vi "Exposure Box.vi"() -> ()   [LabVIEW 2020]
uses:
  epl-vi-lib/Utility VIs/Buttons/KCheckmarkBoolean.ctl
  epl-vi-lib/Utility VIs/Controls/KBackground Gradient/KBackground Gradient.xctl
  Typedefs/TB-Parameters.ctl
  Typedefs/TB-Analysis Parameters.ctl
  Typedefs/TB-Slack State.ctl
  Typedefs/TB-Persistent Data.ctl
  epl-vi-lib/PXI DAQ VIs/AIDI/Typedefs/AIDI-Action.ctl
  epl-vi-lib/PXI DAQ VIs/AODO/Typedefs/AODO-Action.ctl
  Typedefs/TB-State Enum.ctl
  <vilib>/Analysis/baseanly.llb/Mean (DBL).vi
  <vilib>/Analysis/5stat.llb/RMS (DBL).vi
  7ee2e33f-629f-4d1f-82d3-c59bb6443cc8.vi
  <vilib>/Analysis/NI_AALPro.lvlib
  <vilib>/Analysis/NI_AALBase.lvlib
panel:
  out "Exposure":errorcluster
  out "Crown":errorcluster
  in  "Waveform":u16(ring)=2 items=["Noise", "File", "Tone"]
  in  "dB SPL":dbl=100.0
  in  "Duration (min)":dbl=120.0
  in  "Tab Control":enum32{"Tone", "Noise", "File"}(tab)
  in  "Frequency (kHz)":dbl=8.0
  in  "High cutoff (kHz)":dbl=16.0
  in  "Low cutoff (kHz)":dbl=8.0
  in  "refWAV":path caption="Ref"
  in  "WAVfile":path
  in  "Cal Log":path=path "C:/Data/Trauma Box/Trauma Box Calibration Log.txt"
  out "Pistonphone Factor":dbl=102.0 caption="Calibrator Voltage\n(dB rms re 1 uV)"
  in  "B&K Mic Gain":dbl=20.0
  in  "Display":enum32{"Page 1", "Page 2"}(tab)
  out "ma":dbl=99.37258874088361 caption="average" format="%.1f"
  out "Starts":i32
  out "Overload 2":bool caption="Overload"
  in  "Fine Control":dbl(slide) caption="Fine Adjust (dB)" scale=-10.0..6.0
  out "Spectrum":waveform(dbl)(graph)
  out "Waveform":waveform(dbl)(graph)
  out "dB SPL rms":dbl=99.37258874088361 format="%.2f"
  out "Gauge":dbl(knob)=99.37258874088361 scale=80.0..130.0
  out "Elapsed time":string
  out "SPL History":cluster{dbl[], dbl[]}[](graph)
  out "Expected":string="Expected value = 102"
  in  "micCorrFile":path
  in  "Use mic correction":T1 caption="Apply mic frequency correction (if you're unsure, then no)"
  out "Calibration Log":string[][](table)
  out "Overload":bool
  out "Calibrator Voltage\n(dB rms re 1 uV)":dbl=-inf
  out "Pistonphone\nWaveform":dbl[](graph)
  in  "Wizard":T2(tab)
  in  "START":bool
  in  "EXIT":bool
  in  "Use previous":bool
  in  "Remeasure":bool
  in  "Pistonphone measure":bool
  in  "Next":bool
  in  "To Crown adjust":bool
  in  "Start Crown":bool
  in  "Stop Crown":bool
  in  "Start Exposure":bool
  in  "Stop Exposure":bool
  in  "Finished":bool
  in  "User ID":string
  in  "Gradient":dbl(xcontrol)
  # "dB SPL"
  # "Press START to begin\nPress EXIT to quit"
  # "Step 1 Pistonphone correction"
  # "Step 1 Pistonphone correction\n    \n--Put ref mic into pistonphone\n--Make sure B&K gain is correct"
  # "Step 2 Put microphone in cage. It's going to get loud! Close the booth door before continuing."
  # "Step 3 Adjust amplifier until SPL is correct, then hit \"Stop\" button:"
  # "Step 4: Noise Exposure\n1. Put animal(s) in cage\n2. Set duration,\n3. Press START"
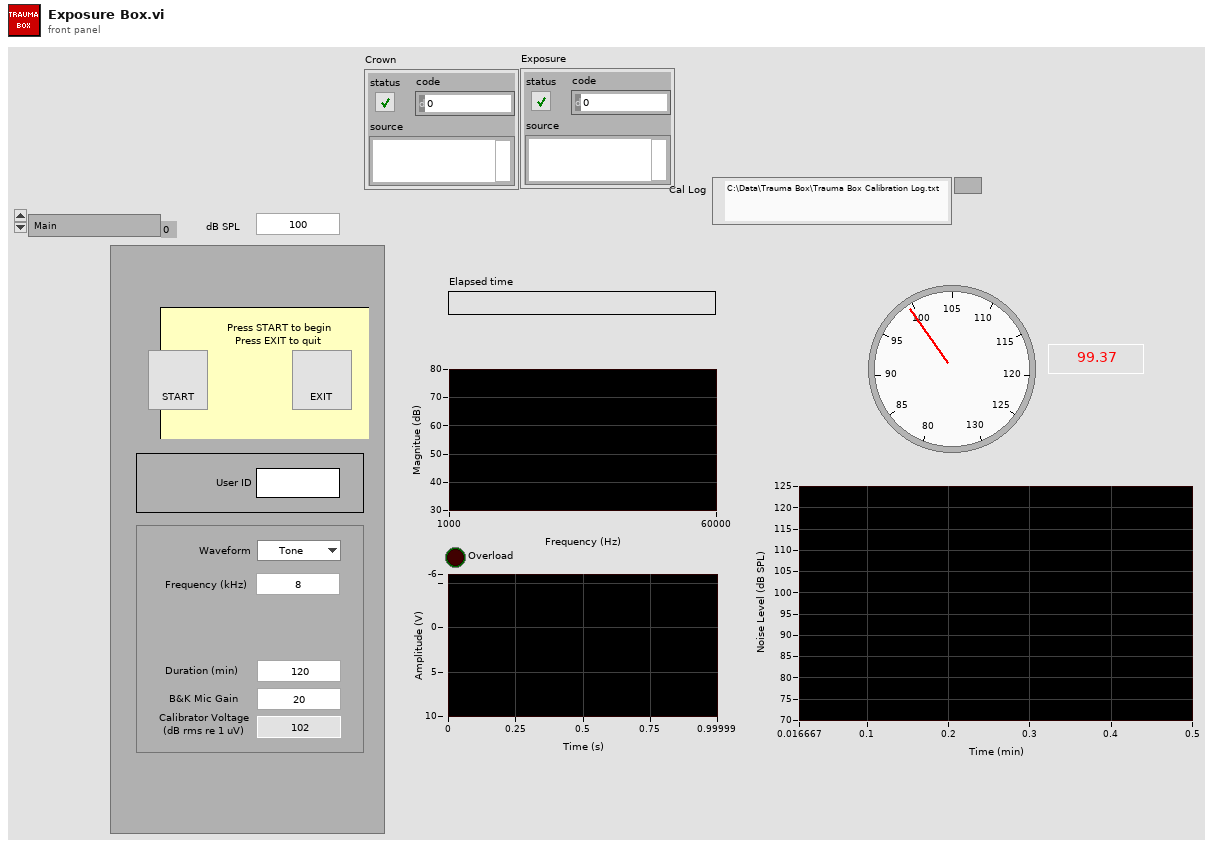
[diagram p1: front panel]
types:
  T1 = typedef "KCheckmarkBoolean.ctl" = bool
  T2 = enum32{"Main", "Pistonphone query", "Pistonphone measure", "Mic in cage", "Adjust Crown", "Animal in cage"}
  T3 = typedef "TB-Persistent Data.ctl" = cluster{"date":string, "cspd scale":dbl}
  T4 = typedef "TB-Slack State.ctl" = cluster{"access_token":string, "bot id":string, "users":cluster{"id":string, "always":bool}[], "chan id":string}
  T5 = typedef "TB-Parameters.ctl" = cluster{"Low cutoff (kHz)":dbl, "High cutoff (kHz)":dbl, "Duration (min)":dbl, "dB SPL":dbl, "Waveform":enum16{"Noise", "File", "Tone"}, "WAVfile":path, "refWav":path, "use mic correction":bool, "micCorrFile":path, "Pistonphone Level (dB SPL)":dbl, "Sampling rate (Hz)":dbl, "Buffer length (s)":dbl, "Stream mic":bool, "Fine adjust":cluster{"Max":dbl, "Min":dbl}, "Mic gain":dbl, "atten":dbl, "Allow Slack":bool, "max starts":i32, "Freq (kHz)":dbl, "Tma (s)":dbl, "Streamed":cluster{"Device":string, "Name":string}[], "Drive":string, "Speaker":string, "Mic":string, "Analysis":T6, "exposeAtten":dbl, "Digital":string}
  T6 = typedef "TB-Analysis Parameters.ctl" = cluster{"Method":enum16{"Default", "Periodogram", "Cross-spectrum"}, "resol (Hz)":dbl, "nfreq":i32, "signal":string}
  T7 = cluster{bool, "Exposure parameters":T5, "Slack":T4}
  T8 = typedef "AODO-Action.ctl" = enum16{"Configure", "Initialize", "Start", "Write", "Clean up", "Init & Start", "Config & Test", "Position", "Set AO Gains", "Zero", "Prime", "Status"}
  T9 = typedef "AIDI-Action.ctl" = enum16{"Configure", "Initialize", "Start", "Read", "Clean up", "Init & Start", "Config & Test", "Position", "Skip"}
  T10 = typedef "TB-Runtime state.ctl" = cluster{"stimfile":T11, "stream mic?":bool, "Fs":dbl, "ID":string, "micCorr":dbl[], "expose":bool, "nacq":i32, "init error":bool, "max starts":i32, "num starts":i32, "Setup":T12, "toneIndex":i32, "LastN":dbl[], "fine":dbl, "stream":refnum<file>, "names":string[], "analysis":T13}
  T11 = typedef "Sound File Refnum.ctl" = refnum<file>
  T12 = typedef "TB-Setup Log.ctl" = cluster{"Pistonphone factor":dbl, "Fine adjust":dbl, "Actual dB SPL":dbl, "CSPD factor":dbl, "Freq":dbl[], "Mag":dbl[]}
  T13 = typedef "TB-Analysis State.ctl" = cluster{"spectra/frame":i32, "pts/spectra":i32, "nfreq":i32, "imic":i32, "isig":i32, "mags":dbl[][], "method":enum16{"Default", "Periodogram", "Cross-spectrum"}, "cspd scale":dbl}
  T14 = typedef "TB-Stimulus State.ctl" = cluster{"filelen":i32, "stimfile":T11, "stimfile?":bool, "Fs":dbl, "Npts":i32, "stimfileend":bool, "atten":dbl, "SigMan":refnum<class "SignalManager.lvclass">, "nbuf":i32, "expose?":bool}
  T15 = typedef "TB-Log.ctl" = cluster{"Slack":T4, "entries":string[]}
  T16 = typedef "TB-Mic Queue.ctl" = refnum<queue>
  T17 = typedef "TB-State Enum.ctl" = enum16{"Main", "Pistonphone query", "Pistonphone measure", "Mic in cage", "Adjust Crown", "Animal in cage"}
  T18 = enum8{"Enabled", "Disabled", "Disabled and Grayed Out"}
  T19 = cluster{"notification":bool, "Parameters out":T5, "Slack":T4}
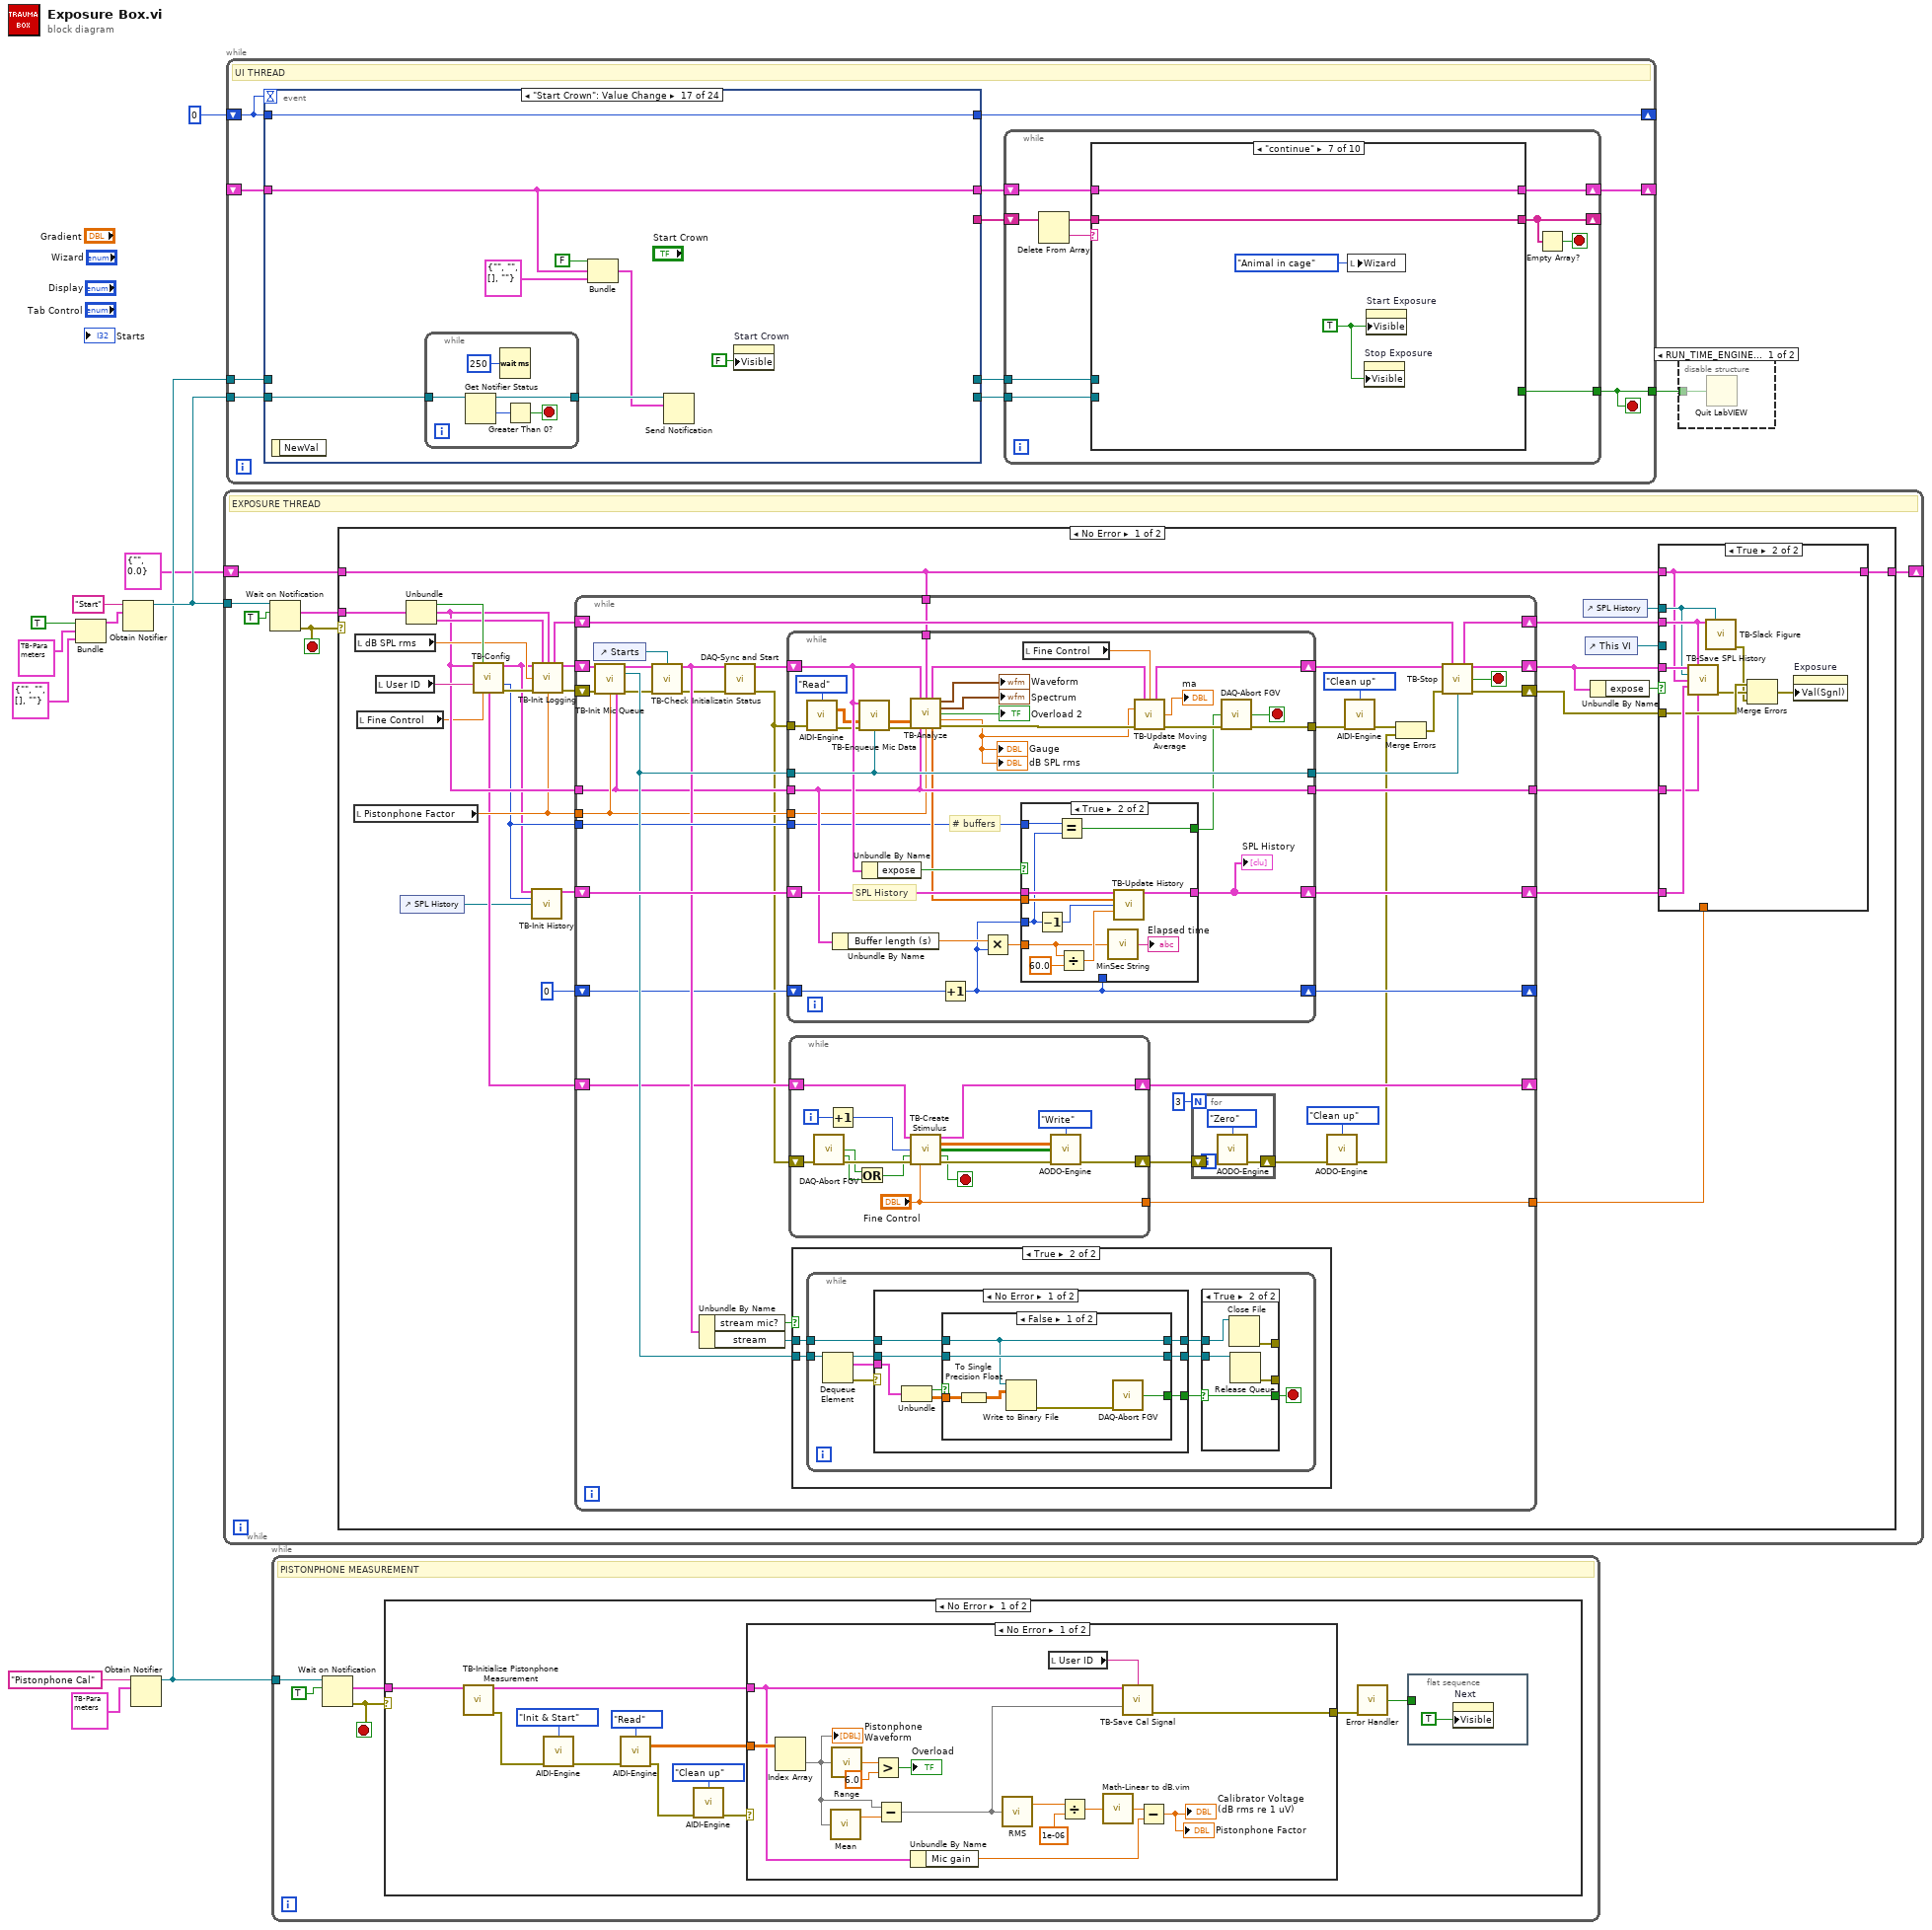
[diagram p0: block diagram]
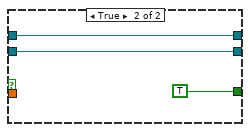
[diagram p5: hidden frame]
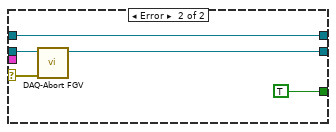
[diagram p6: hidden frame]
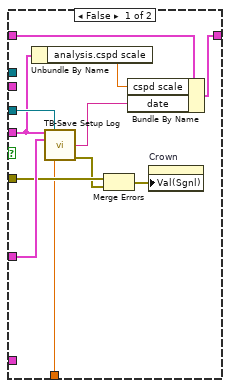
[diagram p7: hidden frame]
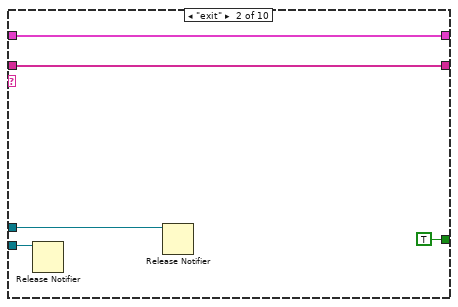
[diagram p10: hidden frame]
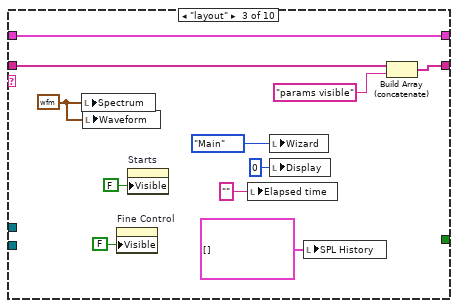
[diagram p11: hidden frame]
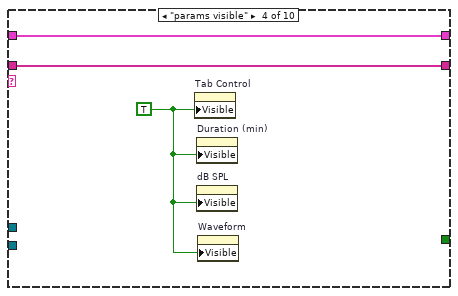
[diagram p12: hidden frame]
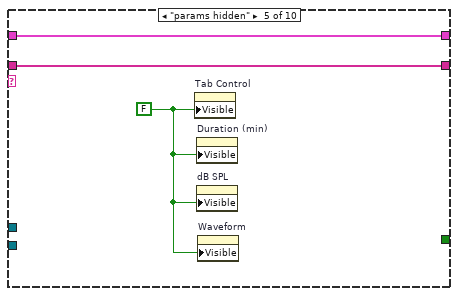
[diagram p13: hidden frame]
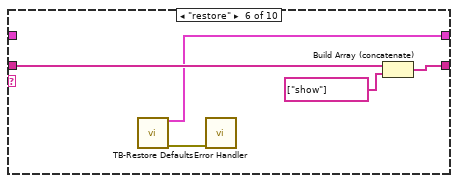
[diagram p14: hidden frame]
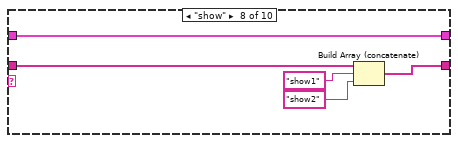
[diagram p15: hidden frame]
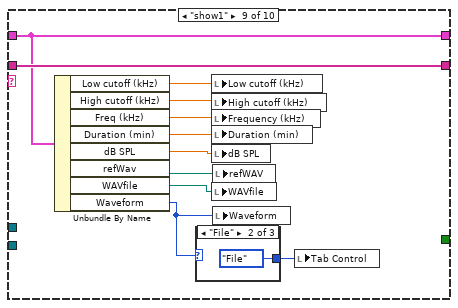
[diagram p16: hidden frame]
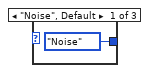
[diagram p17: hidden frame]
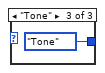
[diagram p18: hidden frame]
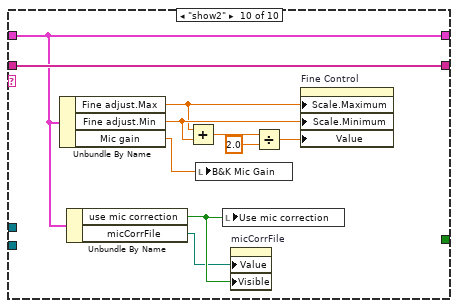
[diagram p19: hidden frame]
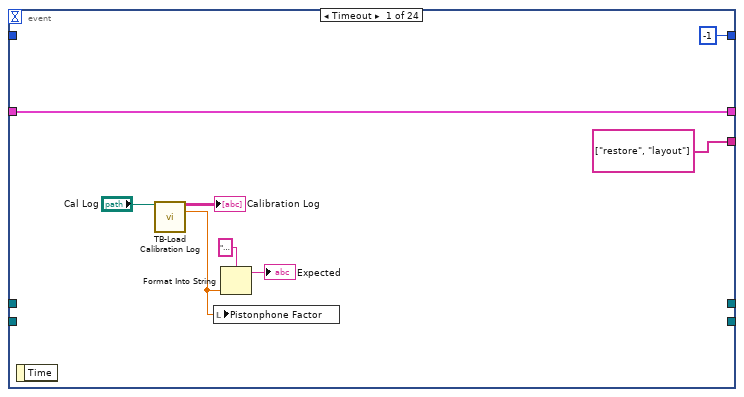
[diagram p20: hidden frame]
diagram:
  n1 = Bundle(TRUE, "Exposure parameters"=T5 {"Low cutoff (kHz)"=0.0, "High cutoff (kHz)"=0.0, "Duration (min)"=0.0, "dB SPL"=0.0, "Waveform"=enum."Noise", "WAVfile"=path "", "refWav"=path "", "use mic correction"=FALSE, "micCorrFile"=path "", "Pistonphone Level (dB SPL)"=0.0, "Sampling rate (Hz)"=0.0, "Buffer length (s)"=0.0, "Stream mic"=FALSE, "Fine adjust"={"Max"=0.0, "Min"=0.0}, "Mic gain"=0.0, "atten"=0.0, "Allow Slack"=FALSE, "max starts"=0, "Freq (kHz)"=8.0, "Tma (s)"=0.0, "Streamed"=[], "Drive"="", "Speaker"="", "Mic"="", "Analysis"={"Method"=enum."Default", "resol (Hz)"=0.0, "nfreq"=0, "signal"=""}, "exposeAtten"=0.0, "Digital"=""}, "Slack"=T4 {"access_token"="", "bot id"="", "users"=[], "chan id"=""}) -> (w4:T7)  [unwired: 1 in]
  n2 = Obtain Notifier(name (unnamed)="Start", notification data type=w4) -> (notifier out=w12:refnum<notifier>)  [unwired: 2 in, 2 out]
  n3 = Obtain Notifier(name (unnamed)="Pistonphone Cal", notification data type=T5 {"Low cutoff (kHz)"=114.0, "High cutoff (kHz)"=100000.0, "Duration (min)"=1.0, "dB SPL"=100.0, "Waveform"=enum."Noise", "WAVfile"=path "", "refWav"=path "", "use mic correction"=FALSE, "micCorrFile"=path "", "Pistonphone Level (dB SPL)"=0.0, "Sampling rate (Hz)"=0.0, "Buffer length (s)"=0.0, "Stream mic"=FALSE, "Fine adjust"={"Max"=0.0, "Min"=0.0}, "Mic gain"=0.0, "atten"=0.0, "Allow Slack"=FALSE, "max starts"=0, "Freq (kHz)"=8.0, "Tma (s)"=0.0, "Streamed"=[], "Drive"="", "Speaker"="", "Mic"="", "Analysis"={"Method"=enum."Default", "resol (Hz)"=0.0, "nfreq"=0, "signal"=""}, "exposeAtten"=0.0, "Digital"=""} ("Exposure parameters")) -> (notifier out=w8:refnum<notifier>)  [unwired: 2 in, 2 out]
  n4 = while {
    tunnel: w12 -> [w17]
    shift-right: [w13] -> _
    shift-left: T3 {"date"="", "cspd scale"=0.0} ("persist") -> [w14]
    stop <- w16 stop-if-true
    # "EXPOSURE THREAD"
    n5 = Wait on Notification(notifier=w17, ignore previous (F)=TRUE) -> (notification=w15:T7, error out=w16:errorcluster)  [unwired: 2 in, 2 out]
    n6 = case shown="No Error" w16 {
      tunnel: w15 -> [w47 _]
      tunnel: w14 -> [w19 w210]
      tunnel: [w20 w210] -> w13
      frame No Error {
        n7 = local read "Pistonphone Factor"() -> (w29:dbl)
        n8 = local read "dB SPL rms"() -> (w37:dbl)
        n9 = local read "Fine Control"() -> (w21:dbl)
        n10 = local read "User ID"() -> (w45:string)
        n11 = control-ref of="SPL History"() -> (w25:refnum<vi>)
        n12 = Unbundle(w47) -> (w46:bool, "Exposure parameters"=w36:T5, "Slack"=w39:T4)
        n13 = call "TB-Config.vi"("Params"=w36, "Exposure?"=w46, "ID"=w45, "Fine adjust (dB)"=w21) -> ("state"=w23:T10, "Num Buffers"=w24:i32, "stimulus state"=w26:T14, "error out"=w41:errorcluster)  [unwired: 8 in]
        n14 = call "TB-Init History.vi"("state"=w23, "Num Buffers"=w24, "XYGraph in"=w25) -> ("history"=w22:cluster{dbl[], dbl[]}[])  [unwired: 12 in]
        n15 = call "TB-Init Logging.vi"("state in"=w23, "Slack"=w39, "Params"=w36, "Level"=w37, "error in (no error)"=w41, "Pistonphone factor"=w29) -> ("Log"=w34:T15, "state out"=w38:T10, "error out"=w40:errorcluster)  [unwired: 7 in]
        n16 = while {
          tunnel: w29 -> [w61]
          tunnel: w24 -> [w81]
          tunnel: w36 -> [w60]
          shift-right: [w82] -> w44
          shift-left: w22 -> [w86]
          shift-right: [w78] -> w42
          shift-left: w40 -> [w77]
          shift-right: [w75] -> w35
          shift-left: w38 -> [w76]
          shift-right: [w73] -> w33
          shift-left: w34 -> [w74]
          shift-right: [w67] -> _
          shift-left: 0 -> [w68]
          shift-right: [w65] -> _
          shift-left: w26 -> [w64]
          tunnel: [w63] -> w30
          tunnel: [w62] -> w28
          tunnel: w19 -> [w50]
          stop <- w69 stop-if-true
          n17 = control-ref of="Starts"() -> (w66:refnum<vi>)
          n18 = call "TB-Init Mic Queue.vi"("state in"=w76, "error in (no error)"=w77, "Pistonphone factor"=w61, "Exposure parameters"=w60) -> ("state out"=w71:T10, "mic queue"=w85:T16, "error out"=w72:errorcluster)  [unwired: 9 in]
          n19 = call "TB-Check Initializatin Status.vi"("state in"=w71, "Starts"=w66, "error in (no error)"=w72) -> ("state out"=w70:T10, "error out"=w53:errorcluster)  [unwired: 11 in]
          n20 = Unbundle By Name(w70) -> ("stream mic?"=w80:bool, "stream"=w84:refnum<file>)
          n21 = call "DAQ-Sync and Start.vi"("error in (no error)"=w53) -> ("error out"=w52:errorcluster)  [unwired: 14 in]
          n22 = while {
            tunnel: w81 -> [w92]
            shift-right: [w118] -> w82
            shift-left: w86 -> [w120]
            tunnel: w61 -> [w99]
            tunnel: w60 -> [w107]
            tunnel: w85 -> [w113]
            tunnel: [w113] -> w83
            shift-right: [w103] -> w79
            shift-left: w70 -> [w110]
            tunnel: [w111] -> w55
            shift-right: [w93] -> w67
            shift-left: w68 -> [w108]
            tunnel: [w107] -> w63
            tunnel: w52 -> [w94]
            tunnel: w50 -> [w90]
            stop <- w112 stop-if-true
            # "# buffers"
            # "SPL History"
            n23 = call "AIDI-Engine.vi"("Action"=AIDI-Action."Read", "error in (no error)"=w94) -> ("AI"=w96:dbl[][], "error out"=w97:errorcluster)  [unwired: 8 in, 4 out]
            n24 = Unbundle By Name(w107) -> ("Buffer length (s)"=w116:dbl)
            n25 = call "TB-Enqueue Mic Data.vi"("state thru"=w110, "AI Waveforms in"=w96, "error in (no error)"=w97, "Queue in"=w113) -> ("AI Waveforms thru"=w115:dbl[][], "error out"=w114:errorcluster)  [unwired: 10 in]
            n26 = Unbundle By Name(w110) -> ("expose"=w109:bool)
            n27 = call "TB-Analyze.vi"("state in"=w110, "persist"=w90, "AI Waveforms"=w115, "error in (no error)"=w114, "Exposure parameters"=w107, "Pistonphone Factor"=w99) -> ("state out"=w104:T10, "waveform"=→"Waveform":waveform(dbl), "spectrum"=→"Spectrum":waveform(dbl), "Overload"=→"Overload 2":bool, "Cal SPL"=w101:dbl, "history values"=w98:dbl[], "error out"=w106:errorcluster)  [unwired: 3 in]
            "Gauge" <- w101
            "dB SPL rms" <- w101
            n28 = Increment(x=w108) -> (x+1=w93:i32)
            n29 = Multiply(x=w116, y=w93) -> (x*y=w121:dbl)
            n30 = case shown="True" w109 {
              tunnel: w121 -> [_ w127]
              tunnel: w120 -> [w123 w132]
              tunnel: [w123 w131] -> w118
              tunnel: w98 -> [_ w130]
              tunnel: w93 -> [_ w125]
              tunnel: w93 -> [_ _]
              tunnel: w92 -> [_ w126]
              tunnel: [_ w124] -> w91
              frame False {
              }
              frame True {
                n31 = Decrement(x=w125) -> (x-1=w129:i32)
                n32 = Equal?(x=w126, y=w125) -> (x = y?=w124:bool)
                n33 = Divide(x=w127, y=60.0) -> (x/y=w128:dbl)
                n34 = call "MinSec String.vi"("Seconds"=w127) -> ("MinSec string"=→"Elapsed time":string)
                n35 = call "TB-Update History.vi"("history in"=w132, "history values"=w130, "Index"=w129, "Time"=w128) -> ("history out"=w131:cluster{dbl[], dbl[]}[])  [unwired: 11 in]
              }
            }
            "SPL History" <- w118
            n36 = local read "Fine Control"() -> (w100:dbl)
            n37 = call "TB-Update Moving Average.vi"("state in"=w104, "fine"=w100, "SPL"=w101, "error in (no error)"=w106) -> ("state out"=w103:T10, "moving average"=→"ma":dbl, "error out"=w105:errorcluster)  [unwired: 9 in]
            n38 = call "DAQ-Abort FGV.vi"("Finished"=w91, "error in (no error)"=w105) -> ("Stop"=w112:bool, "Errors"=w111:errorcluster)  [unwired: 11 in, 1 out]
          }
          n39 = while {
            shift-right: [w148] -> w51
            shift-left: w52 -> [w143]
            shift-right: [w146] -> w65
            shift-left: w64 -> [w147]
            tunnel: ["Fine Control"] -> w62
            i -> [w144]
            stop <- w140 stop-if-true
            n40 = call "DAQ-Abort FGV.vi"("error in (no error)"=w143) -> ("Stop"=w139:bool, "Was aborted"=w138:bool, "Errors"=w142:errorcluster)  [unwired: 12 in]
            n41 = Increment(x=w144) -> (x+1=w141:i32)
            n42 = Or(x=w139, y=w138) -> (x .or. y?=w137:bool)
            n43 = call "TB-Create Stimulus.vi"("state"=w147, "Num"=w141, "quit"=w137, "error in (no error)"=w142, "Fine adjust (dB)"="Fine Control") -> ("state out"=w146:T14, "stimulus"=w136:dbl[][], "digital"=w135:bool[][], "finished"=w140:bool, "error out"=w149:errorcluster)  [unwired: 6 in]
            n44 = call "AODO-Engine.vi"("Action"=AODO-Action."Write", "AO"=w136, "DO"=w135, "error in (no error)"=w149) -> ("error out"=w148:errorcluster)  [unwired: 6 in, 5 out]
          }
          n45 = case shown="True" w80 {
            tunnel: w85 -> [_ w152]
            tunnel: w84 -> [_ w151]
            frame False {
            }
            frame True {
              n46 = while {
                tunnel: w152 -> [w161]
                tunnel: w151 -> [w155]
                stop <- w156 stop-if-true
                n47 = Dequeue Element(queue=w161) -> (queue out=w158:T16, element=w159:cluster{bool, dbl[][]}, error out=w160:errorcluster)  [unwired: 2 in, 1 out]
                n48 = case shown="No Error" w160 {
                  selector: w160 -> [_ w185]
                  tunnel: w159 -> [w175 _]
                  tunnel: [w173 TRUE ("status")] -> w157
                  tunnel: w158 -> [w171 w186]
                  tunnel: w155 -> [w170 w187]
                  tunnel: [w169 w187] -> w154
                  tunnel: [w168 w186] -> w153
                  frame No Error {
                    n49 = Unbundle(w175) -> (w174:bool, w172:dbl[][])
                    n50 = case shown="False" w174 {
                      tunnel: [w180 TRUE ("status")] -> w173
                      tunnel: w172 -> [w177 _]
                      tunnel: w171 -> [w181 w182]
                      tunnel: w170 -> [w179 w183]
                      tunnel: [w179 w183] -> w169
                      tunnel: [w181 w182] -> w168
                      frame False {
                        n51 = To Single Precision Float(number=w177) -> (single precision float=w176:sgl[][])
                        n52 = Write to Binary File(file (use dialog)=w179, data=w176) -> (error out=w178:errorcluster)  [unwired: 4 in, 2 out]
                        n53 = call "DAQ-Abort FGV.vi"("error in (no error)"=w178) -> ("Stop"=w180:bool)  [unwired: 12 in, 2 out]
                      }
                      frame True {
                      }
                    }
                  }
                  frame Error {
                    n54 = call "DAQ-Abort FGV.vi"("error in (no error)"=w185) -> ()  [unwired: 12 in, 3 out]
                  }
                }
                n55 = case shown="True" w157 {
                  selector: w157 -> [w162 w167]
                  tunnel: [w162 w167] -> w156
                  tunnel: w154 -> [_ w164]
                  tunnel: w153 -> [_ w166]
                  tunnel: [_ w165] -> _
                  tunnel: [_ w163] -> _
                  frame False {
                  }
                  frame True {
                    n56 = Close File(refnum=w164) -> (error out=w163:errorcluster)  [unwired: 1 in, 1 out]
                    n57 = Release Queue(queue=w166) -> (error out=w165:errorcluster)  [unwired: 2 in, 2 out]
                  }
                }
              }
            }
          }
          n58 = for {
            N: 3 -> [_]
            shift-right: [w87] -> w49
            shift-left: w51 -> [w89]
            n59 = call "AODO-Engine.vi"("Action"=AODO-Action."Zero", "error in (no error)"=w89) -> ("error out"=w87:errorcluster)  [unwired: 8 in, 5 out]
          }
          n60 = call "AODO-Engine.vi"("Action"=AODO-Action."Clean up", "error in (no error)"=w49) -> ("error out"=w57:errorcluster)  [unwired: 8 in, 5 out]
          n61 = call "AIDI-Engine.vi"("Action"=AIDI-Action."Clean up", "error in (no error)"=w55) -> ("error out"=w56:errorcluster)  [unwired: 8 in, 5 out]
          n62 = Merge Errors(w56, w57) -> (w54:errorcluster)
          n63 = call "TB-Stop.vi"("state in"=w79, "Log in"=w74, "error in (no error)"=w54, "Queue in"=w83) -> ("Log out"=w73:T15, "state out"=w75:T10, "Finished"=w69:bool, "error out"=w78:errorcluster)  [unwired: 8 in]
        }
        n64 = control-ref of="SPL History"() -> (w31:refnum<vi>)
        n65 = control-ref of="This VI"() -> (w27:refnum<vi>)
        n66 = Unbundle By Name(w35) -> ("expose"=w43:bool)
        n67 = case shown="True" w43 {
          tunnel: w44 -> [_ w209]
          tunnel: w35 -> [w190 w208]
          tunnel: w42 -> [w198 w207]
          tunnel: w33 -> [_ w203]
          tunnel: w31 -> [_ w202]
          tunnel: w30 -> [w199 w201]
          tunnel: w28 -> [w195 _]
          tunnel: w27 -> [w194 _]
          tunnel: w19 -> [w193 w200]
          tunnel: [w191 w200] -> w20
          frame False {
            n68 = Unbundle By Name(w190) -> ("analysis.cspd scale"=w189:dbl)
            n69 = call "TB-Save Setup Log.vi"("State"=w190, "VI ref"=w194, "Exposure parameters"=w199, "Fine Control"=w195) -> ("date/time string"=w192:string, "error out"=w196:errorcluster)  [unwired: 10 in]
            n70 = Merge Errors(w198, w196) -> (w197:errorcluster)
            n71 = Bundle By Name(cluster=w193, "cspd scale"=w189, "date"=w192) -> (w191:T3)
            n72 = property on="Crown" class="Clust (strict)"("Val(Sgnl)"=w197) -> ()  [unwired: 2 in, 2 out]
          }
          frame True {
            n73 = call "TB-Save SPL History.vi"("state"=w208, "Log in"=w203, "XYGraph in"=w202, "persistent"=w200, "history"=w209, "Exposure parameters"=w201) -> ("error out"=w205:errorcluster)  [unwired: 9 in]
            n74 = call "TB-Slack Figure.vi"("Log"=w203, "XYGraph in"=w202) -> ("error out"=w204:errorcluster)  [unwired: 13 in]
            n75 = Merge Errors(w207, w205, w204) -> (w206:errorcluster)
            n76 = property on="Exposure" class="Clust (strict)"("Val(Sgnl)"=w206) -> ()  [unwired: 2 in, 2 out]
          }
        }
      }
      frame Error {
      }
    }
  }
  n77 = while {
    tunnel: w12 -> [w221]
    shift-right: [w220] -> _
    shift-left: 0 -> [w217]
    tunnel: w8 -> [w219]
    tunnel: [w211] -> w7
    shift-right: [w212] -> _
    shift-left: _ -> [w218]
    stop <- w211 stop-if-true
    # "UI THREAD"
    n78 = event shown="[16] \"Start Crown\": Value Change" {
      selector: _ -> [_ _ _ _ _ _ _ _ _ _ _ _ _ _ _ _ _ _ _ _ _ _ _ _]
      dyn-events: _ -> [_ _ _ _ _ _ _ _ _ _ _ _ _ _ _ _ _ _ _ _ _ _ _ _]
      timeout: w217 -> [_ _ _ _ _ _ _ _ _ _ _ _ _ _ _ _ _ _ _ _ _ _ _ _]
      tunnel: w221 -> [_ w302 w309 _ _ _ _ _ _ _ _ _ _ _ _ w411 w419 _ w453 _ _ w474 _ _]
      tunnel: [_ w302 w309 _ _ _ _ _ _ _ _ _ _ _ _ _ _ _ _ _ _ w474 _ _] -> w214
      tunnel: [-1 w305 w313 w340 w346 w352 w355 w360 w368 w369 w374 w381 w385 w391 w394 w404 w415 w428 w436 w465 w467 w471 w478 w484] -> w220
      tunnel: w219 -> [_ w303 w310 _ _ _ _ _ _ _ _ _ _ w392 _ _ _ _ _ _ _ w473 _ _]
      tunnel: [_ w303 w310 _ _ _ _ _ _ _ _ _ _ _ _ _ _ _ _ _ _ w473 _ _] -> w215
      tunnel: [w298 w306 w311 w341 w349 w353 w358 w363 w366 w372 w375 w382 w386 w390 w395 w401 w416 w429 w434 w466 w468 w472 w477 w483] -> w213
      tunnel: w218 -> [w298 w306 w314 w342 w350 w354 w359 w364 w367 w373 w375 w382 w386 w390 w395 w401 w416 w429 w434 w466 w468 w472 w477 w483]
      tunnel: w217 -> [_ w305 w313 w340 w346 w352 w355 w360 w368 w369 w374 w381 w385 w391 w394 w404 w415 w428 w436 w465 w467 w471 w478 w484]
      tunnel: [string[] ["restore", "layout"] string[] ["exit"] w312 _ _ _ _ _ _ _ _ _ string[] ["params hidden"] _ string[] ["params visible"] _ _ _ _ _ _ string[] ["exit"] _ _] -> w216
      event Timeout {
        n79 = event-data() -> ()  [unwired: 1 in, 1 out]
        n80 = call "TB-Load Calibration Log.vi"("Cal Log"="Cal Log") -> ("Log"=→"Calibration Log":string[][], "mean value"=w296:dbl)  [unwired: 13 in]
        n81 = local write "Pistonphone Factor"(w296) -> ()
        n82 = Format Into String(format string="Expected value = %d", w296) -> (resulting string=→"Expected":string)  [unwired: 2 in, 1 out]
      }
      event Panel Close? {
        n83 = event-data() -> ()  [unwired: 1 in, 1 out]
        n84 = event-data("Discard?"=TRUE) -> ()  [unwired: 1 in, 1 out]
      }
      event Menu Selection (User) {
        n85 = event-data() -> ("ItemTag"=w315:string)  [unwired: 1 in]
        n86 = case shown="\"mmFileContinue\"" w315 {
          tunnel: [_ _ w324 _ _ _ _] -> w308
          tunnel: w314 -> [w316 w317 w321 w330 w332 w334 w336]
          tunnel: [w316 w317 w320 w330 w332 w334 w337] -> w311
          tunnel: [_ string[] ["restore"] _ string[] ["restore", "layout"] string[] ["continue"] string[] ["exit"] _] -> w312
          frame "", Default {
          }
          frame "mmFileRestore" {
          }
          frame "mmFileSave" {
            n87 = property on="Fine Control" class="Slide (strict)"() -> ("Scale.Maximum"=w323:dbl, "Scale.Minimum"=w322:dbl)  [unwired: 2 in, 2 out]
            n88 = Bundle By Name(cluster=w321, "Fine adjust.Max"=w323, "Fine adjust.Min"=w322) -> (w320:T5)
            n89 = call "Default Config File Path.vi"() -> ("Default config file name"=w326:path)
            n90 = call "Write Anything.vi"("Section Name (Name of \"Anything\")"="Params" ("Section Name (Name of \"Anything\")"), "Anything"=w320, "Path (dialog)"=w326) -> ("Error Out"=w325:errorcluster)  [unwired: 7 in, 1 out]
            n91 = case shown="No Error" w325 {
              selector: w325 -> [_ w328]
              tunnel: [_ w328] -> w324
              frame No Error {
                n92 = One Button Dialog(message="Defaults saved.") -> ()  [unwired: 1 in, 1 out]
              }
              frame Error {
              }
            }
          }
          frame "mmFileRestart" {
          }
          frame "mmFileContinue" {
          }
          frame "mmFileExit" {
          }
          frame "mmEditOptions" {
            n93 = control-ref of="This VI"() -> (w335:refnum<vi>)
            n94 = call "TB-Options Dialog.vi"("Parameters in"=w336, "Parent VI"=w335) -> ("Parameters out"=w337:T5)  [unwired: 12 in, 1 out]
          }
        }
        n95 = call "Error Handler.vi"("error in (no error)"=w308) -> ()  [unwired: 12 in, 3 out]
      }
      event "Waveform": Value Change {
        n96 = event-data() -> ()  [unwired: 1 in, 1 out]
        n97 = case shown="1" "Waveform" {
          tunnel: [enum32{"Tone", "Noise", "File"}."Noise" ("Tab Control") enum32{"Tone", "Noise", "File"}."File" ("Tab Control") enum32{"Tone", "Noise", "File"}."Tone" ("Tab Control")] -> w339
          frame 0, Default {
          }
          frame 1 {
          }
          frame 2 {
          }
        }
        n98 = local write "Tab Control"(w339) -> ()
        n99 = Bundle By Name(cluster=w342, "Waveform"="Waveform") -> (w341:T5)
      }
      event "Low cutoff (kHz)", "High cutoff (kHz)": Value Change {
        n100 = event-data() -> ()  [unwired: 1 in, 1 out]
        n101 = Bundle By Name(cluster=w350, "Low cutoff (kHz)"="Low cutoff (kHz)", "High cutoff (kHz)"="High cutoff (kHz)") -> (w349:T5)
      }
      event "Frequency (kHz)": Value Change {
        n102 = event-data() -> ()  [unwired: 1 in, 1 out]
        n103 = Bundle By Name(cluster=w354, "Freq (kHz)"="Frequency (kHz)") -> (w353:T5)
      }
      event "WAVfile", "refWAV": Value Change {
        n104 = event-data() -> ()  [unwired: 1 in, 1 out]
        n105 = Bundle By Name(cluster=w359, "WAVfile"="WAVfile", "refWav"="refWAV") -> (w358:T5)
      }
      event "micCorrFile": Value Change {
        n106 = event-data() -> ()  [unwired: 1 in, 1 out]
        n107 = Bundle By Name(cluster=w364, "use mic correction"="Use mic correction", "micCorrFile"="micCorrFile") -> (w363:T5)
        n108 = property on="micCorrFile" class="Path"("Visible"="Use mic correction") -> ()  [unwired: 2 in, 2 out]
      }
      event "B&K Mic Gain": Value Change {
        n109 = event-data() -> ()  [unwired: 1 in, 1 out]
        n110 = Bundle By Name(cluster=w367, "Mic gain"="B&K Mic Gain") -> (w366:T5)
      }
      event "Duration (min)", "dB SPL": Value Change {
        n111 = event-data() -> ()  [unwired: 1 in, 1 out]
        n112 = Bundle By Name(cluster=w373, "Duration (min)"="Duration (min)", "dB SPL"="dB SPL") -> (w372:T5)
      }
      event "START": Value Change {
        n113 = event-data() -> ()  [unwired: 1 in, 1 out]
        n114 = Empty String/Path?(string/path="User ID") -> (empty?=w376:bool)
        n115 = case shown="False" w376 {
          frame False {
            n116 = property on="Starts" class="DigNum (strict)"("Visible"=FALSE) -> ()  [unwired: 2 in, 2 out]
            n117 = local write "Wizard"(TB-State_Enum."Pistonphone query" ("State")) -> ()
          }
          frame True {
            n118 = One Button Dialog(message="Please enter a User ID (for bookkeeping purposes).") -> ()  [unwired: 1 in, 1 out]
          }
        }
      }
      event "Use previous": Value Change {
        n119 = event-data() -> ()  [unwired: 1 in, 1 out]
        n120 = local write "Wizard"(TB-State_Enum."Mic in cage" ("State")) -> ()
      }
      event "Remeasure": Value Change {
        n121 = event-data() -> ()  [unwired: 1 in, 1 out]
        n122 = property on="Next" class="Bool"("Visible"=FALSE) -> ()  [unwired: 2 in, 2 out]
        n123 = local write "Display"(1) -> ()
        n124 = local write "Wizard"(TB-State_Enum."Pistonphone measure" ("State")) -> ()
      }
      event "Pistonphone measure": Value Change {
        n125 = event-data() -> ()  [unwired: 1 in, 1 out]
        n126 = Send Notification(notification=w390, notifier=w392) -> ()  [unwired: 1 in, 2 out]
      }
      event "Next": Value Change {
        n127 = event-data() -> ()  [unwired: 1 in, 1 out]
        n128 = local write "Wizard"(TB-State_Enum."Mic in cage" ("State")) -> ()
        n129 = local write "Display"(0) -> ()
      }
      event "To Crown adjust": Value Change {
        n130 = event-data() -> ()  [unwired: 1 in, 1 out]
        n131 = property on="Fine Control" class="Slide (strict)"("Visible"=TRUE, "Value"=0.0 ("Fine Control")) -> (error out=w406:errorcluster)  [unwired: 2 in, 1 out]
        n132 = local write "Elapsed time"("" ("Elapsed time")) -> ()
        n133 = local write "Wizard"(TB-State_Enum."Adjust Crown" ("State")) -> ()
        n134 = Bundle("notification"=FALSE, "Parameters out"=w401, "Slack"=T4 {"access_token"="", "bot id"="", "users"=[], "chan id"=""}) -> (w403:T19)  [unwired: 1 in]
        n135 = Send Notification(notification=w403, notifier=w411, error in (no error)=w406) -> ()  [unwired: 2 out]
        n136 = property on="Start Crown" class="Bool"("Visible"=FALSE) -> ()  [unwired: 2 in, 2 out]
        n137 = property on="Stop Crown" class="Bool"("DisabledEnum"=T18."Enabled" ("Disabled")) -> ()  [unwired: 2 in, 2 out]
        n138 = Unbundle By Name(w401) -> ("Tma (s)"=w400:dbl)
        n139 = Greater Than 0?(x=w400) -> (x > 0?=w399:bool)
        n140 = property on="ma" class="DigNum (strict)"("Visible"=w399) -> ()  [unwired: 2 in, 2 out]
      }
      event "Start Crown": Value Change {
        n141 = event-data() -> ()  [unwired: 1 in, 1 out]
        n142 = while {
          tunnel: w419 -> [w425]
          tunnel: [w421] -> w418
          stop <- w423 stop-if-true
          n143 = Get Notifier Status(notifier=w425) -> (notifier out=w421:refnum<notifier>, # waiting=w424:i32)  [unwired: 1 in, 3 out]
          n144 = Wait (ms)(milliseconds to wait=u32 250) -> ()  [unwired: 1 out]
          n145 = Greater Than 0?(x=w424) -> (x > 0?=w423:bool)
        }
        n146 = Bundle("notification"=FALSE, "Parameters out"=w416, "Slack"=T4 {"access_token"="", "bot id"="", "users"=[], "chan id"=""}) -> (w414:T19)  [unwired: 1 in]
        n147 = Send Notification(notification=w414, notifier=w418) -> ()  [unwired: 1 in, 2 out]
        n148 = property on="Start Crown" class="Bool"("Visible"=FALSE) -> ()  [unwired: 2 in, 2 out]
      }
      event "Stop Crown": Value Change {
        n149 = event-data() -> ()  [unwired: 1 in, 1 out]
        n150 = property on="Stop Crown" class="Bool"("DisabledEnum"=T18."Disabled and Grayed Out" ("Disabled")) -> ()  [unwired: 2 in, 2 out]
        n151 = call "DAQ-Abort FGV.vi"("Action"=enum16{"Default", "Init", "Abort", "1st error"}."Abort") -> ()  [unwired: 12 in, 3 out]
      }
      event "Start Exposure": Value Change {
        n152 = event-data() -> ("CtlRef"=w431:refnum<vi>)  [unwired: 1 in]
        n153 = local read "Pistonphone Factor"() -> (w447:dbl)
        n154 = Get Date/Time In Seconds() -> (seconds since 1Jan1904=w448:timestamp)
        n155 = local read "User ID"() -> (w449:string)
        n156 = local read "Cal Log"() -> (w439:path)
        n157 = Get Date/Time String(seconds (now)=w448) -> (date string=w446:string)  [unwired: 2 in, 1 out]
        n158 = Strip Path(path=w439) -> (stripped path=w441:path)  [unwired: 1 out]
        n159 = property on="Start Exposure" class="Bool"("Visible"=FALSE) -> ()  [unwired: 2 in, 2 out]
        n160 = call "FileIO-File or Folder Exists.vi"("path"=w441) -> ("Directory?"=w440:bool, "dup path"=w438:path)  [unwired: 7 in, 2 out]
        n161 = Format Into String(format string="%s\t%s\t%.2f\n", w449, w446, w447) -> (resulting string=w450:string)  [unwired: 2 in, 1 out]
        n162 = case shown="False" w440 {
          tunnel: w438 -> [w458 _]
          tunnel: [w457 _] -> w437
          frame False {
            n163 = Create Folder(path (use dialog)=w458) -> (error out=w457:errorcluster)  [unwired: 2 in, 2 out]
          }
          frame True {
          }
        }
        n164 = Unbundle By Name(w434) -> ("Duration (min)"=w443:dbl)
        n165 = call "Append to Text File.vi"("file path"=w439, "text"=w450, "error in (no error)"=w437) -> ("error out"=w444:errorcluster)  [unwired: 11 in, 1 out]
        n166 = property on="SPL History" class="XYGraph (strict)"(error in=w444, "XScale.Maximum"=w443) -> (error out=w445:errorcluster)  [unwired: 1 in, 1 out]
        n167 = Unbundle By Name(w434) -> ("Allow Slack"=w432:bool)
        n168 = property on="ma" class="DigNum (strict)"("Visible"=FALSE) -> ()  [unwired: 2 in, 2 out]
        n169 = while {
          tunnel: w453 -> [w463]
          tunnel: [w459] -> w454
          tunnel: w445 -> [_]
          stop <- w461 stop-if-true
          n170 = Wait (ms)(milliseconds to wait=u32 250) -> ()  [unwired: 1 out]
          n171 = Get Notifier Status(notifier=w463) -> (notifier out=w459:refnum<notifier>, # waiting=w462:i32)  [unwired: 1 in, 3 out]
          n172 = Greater Than 0?(x=w462) -> (x > 0?=w461:bool)
        }
        n173 = call "TB-Init Slack.vi"("Allow Slack"=w432, "CtlRef"=w431) -> ("Slack"=w433:T4)  [unwired: 13 in]
        n174 = property on="Stop Exposure" class="Bool"("Visible"=TRUE) -> ()  [unwired: 2 in, 2 out]
        n175 = Bundle("notification"=TRUE, "Parameters out"=w434, "Slack"=w433) -> (w435:T19)  [unwired: 1 in]
        n176 = property on="Fine Control" class="Slide (strict)"("Visible"=FALSE) -> ()  [unwired: 2 in, 2 out]
        n177 = Send Notification(notification=w435, notifier=w454) -> ()  [unwired: 1 in, 2 out]
      }
      event "Stop Exposure": Value Change {
        n178 = event-data() -> ()  [unwired: 1 in, 1 out]
        n179 = call "DAQ-Abort FGV.vi"("Action"=enum16{"Default", "Init", "Abort", "1st error"}."Abort") -> ()  [unwired: 12 in, 3 out]
      }
      event "Finished": Value Change {
        n180 = event-data() -> ()  [unwired: 1 in, 1 out]
        n181 = local write "Wizard"(TB-State_Enum."Main" ("State")) -> ()
      }
      event "EXIT": Value Change {
        n182 = event-data() -> ()  [unwired: 1 in, 1 out]
      }
      event "Crown": Value Change {
        n183 = event-data() -> ("NewVal"=w476:errorcluster, "NewVal.status"=w475:bool)  [unwired: 1 in]
        n184 = call "Error Handler.vi"("error in (no error)"=w476) -> ()  [unwired: 12 in, 3 out]
        n185 = property on="Start Crown" class="Bool"("Visible"=w475) -> ()  [unwired: 2 in, 2 out]
        n186 = case shown="False" w475 {
          frame False {
            w480 = TRUE ("Visible")
            n187 = property on="Start Exposure" class="Bool"("Visible"=w480) -> ()  [unwired: 2 in, 2 out]
            n188 = property on="Stop Exposure" class="Bool"("Visible"=w480) -> ()  [unwired: 2 in, 2 out]
            n189 = local write "Wizard"(TB-State_Enum."Animal in cage" ("State")) -> ()
          }
          frame True {
          }
        }
      }
      event "Exposure": Value Change {
        n190 = event-data() -> ("NewVal"=w481:errorcluster)  [unwired: 1 in]
        n191 = call "Error Handler.vi"("error in (no error)"=w481) -> ()  [unwired: 12 in, 3 out]
        n192 = property on="Stop Exposure" class="Bool"("Visible"=FALSE) -> ()  [unwired: 2 in, 2 out]
      }
    }
    n193 = while {
      shift-right: [w228] -> _
      shift-left: w216 -> [w231]
      tunnel: w215 -> [w226]
      tunnel: w214 -> [w225]
      shift-right: [w223] -> w212
      shift-left: w213 -> [w224]
      tunnel: [w222] -> w211
      stop <- w227 stop-if-true
      n194 = Delete From Array(array=w231) -> (deleted portion=w229:string, array with subset deleted=w230:string[])  [unwired: 2 in]
      n195 = case shown="\"continue\"" w229 {
        tunnel: w230 -> [w233 w238 w249 w252 w255 w260 w264 w269 w280 w293]
        tunnel: [w233 w238 w242 w252 w255 w257 w264 w267 w280 w293] -> w228
        tunnel: w226 -> [_ w237 _ _ _ _ _ _ _ _]
        tunnel: w225 -> [_ w236 _ _ _ _ _ _ _ _]
        tunnel: w224 -> [w232 w235 w248 w251 w254 _ w263 w268 w273 w284]
        tunnel: [w232 w235 w248 w251 w254 w258 w263 w268 w273 w284] -> w223
        tunnel: [_ TRUE _ _ _ _ _ _ _ _] -> w222
        frame "", Default {
        }
        frame "exit" {
          n196 = Release Notifier(notifier=w236) -> ()  [unwired: 2 in, 3 out]
          n197 = Release Notifier(notifier=w237) -> ()  [unwired: 2 in, 3 out]
        }
        frame "layout" {
          w247 = waveform(dbl) {"t0"=timestamp(0 s since 1904-01-01), "dt"=1.0, "Y"=[]} ("Spectrum")
          n198 = local write "Spectrum"(w247) -> ()
          n199 = local write "Waveform"(w247) -> ()
          n200 = property on="Fine Control" class="Slide (strict)"("Visible"=FALSE) -> ()  [unwired: 2 in, 2 out]
          n201 = property on="Starts" class="DigNum (strict)"("Visible"=FALSE) -> ()  [unwired: 2 in, 2 out]
          n202 = local write "Elapsed time"("") -> ()
          n203 = local write "Wizard"(TB-State_Enum."Main" ("State")) -> ()
          n204 = local write "Display"(0) -> ()
          n205 = local write "SPL History"(cluster{dbl[], dbl[]}[] [] ("SPL History")) -> ()
          n206 = Build Array (concatenate)(w249, "params visible") -> (w242:string[])
        }
        frame "params visible" {
          w250 = TRUE
          n207 = property on="Tab Control" class="TabCtl (strict)"("Visible"=w250) -> ()  [unwired: 2 in, 2 out]
          n208 = property on="Duration (min)" class="DigNum (strict)"("Visible"=w250) -> ()  [unwired: 2 in, 2 out]
          n209 = property on="dB SPL" class="DigNum (strict)"("Visible"=w250) -> ()  [unwired: 2 in, 2 out]
          n210 = property on="Waveform" class="Ring (strict)"("Visible"=w250) -> ()  [unwired: 2 in, 2 out]
        }
        frame "params hidden" {
          w253 = FALSE
          n211 = property on="Tab Control" class="TabCtl (strict)"("Visible"=w253) -> ()  [unwired: 2 in, 2 out]
          n212 = property on="Duration (min)" class="DigNum (strict)"("Visible"=w253) -> ()  [unwired: 2 in, 2 out]
          n213 = property on="dB SPL" class="DigNum (strict)"("Visible"=w253) -> ()  [unwired: 2 in, 2 out]
          n214 = property on="Waveform" class="Ring (strict)"("Visible"=w253) -> ()  [unwired: 2 in, 2 out]
        }
        frame "restore" {
          n215 = call "TB-Restore Defaults.vi"() -> ("Exposure parameters out"=w258:T5, "error out"=w259:errorcluster)  [unwired: 14 in]
          n216 = call "Error Handler.vi"("error in (no error)"=w259) -> ()  [unwired: 12 in, 3 out]
          n217 = Build Array (concatenate)(w260, string[] ["show"]) -> (w257:string[])
        }
        frame "continue" {
          w261 = TRUE
          n218 = local write "Wizard"(T2."Animal in cage" ("Wizard")) -> ()
          n219 = property on="Stop Exposure" class="Bool"("Visible"=w261) -> ()  [unwired: 2 in, 2 out]
          n220 = property on="Start Exposure" class="Bool"("Visible"=w261) -> ()  [unwired: 2 in, 2 out]
        }
        frame "show" {
          n221 = Build Array (concatenate)(w269, "show1", "show2") -> (w267:string[])
        }
        frame "show1" {
          n222 = Unbundle By Name(w273) -> ("Low cutoff (kHz)"=w274:dbl, "High cutoff (kHz)"=w275:dbl, "Freq (kHz)"=w270:dbl, "Duration (min)"=w276:dbl, "dB SPL"=w277:dbl, "refWav"=w279:path, "WAVfile"=w278:path, "Waveform"=w272:enum16{"Noise", "File", "Tone"})
          n223 = case shown="\"File\"" w272 {
            tunnel: [enum32{"Tone", "Noise", "File"}."Noise" ("Tab Control") enum32{"Tone", "Noise", "File"}."File" ("Tab Control") enum32{"Tone", "Noise", "File"}."Tone" ("Tab Control")] -> w271
            frame "Noise", Default {
            }
            frame "File" {
            }
            frame "Tone" {
            }
          }
          n224 = local write "Low cutoff (kHz)"(w274) -> ()
          n225 = local write "High cutoff (kHz)"(w275) -> ()
          n226 = local write "Frequency (kHz)"(w270) -> ()
          n227 = local write "Duration (min)"(w276) -> ()
          n228 = local write "dB SPL"(w277) -> ()
          n229 = local write "WAVfile"(w278) -> ()
          n230 = local write "refWAV"(w279) -> ()
          n231 = local write "Waveform"(w272) -> ()
          n232 = local write "Tab Control"(w271) -> ()
        }
        frame "show2" {
          n233 = Unbundle By Name(w284) -> ("Fine adjust.Max"=w288:dbl, "Fine adjust.Min"=w289:dbl, "Mic gain"=w292:dbl)
          n234 = Unbundle By Name(w284) -> ("use mic correction"=w286:bool, "micCorrFile"=w285:path)
          n235 = Add(x=w288, y=w289) -> (x+y=w287:dbl)
          n236 = local write "B&K Mic Gain"(w292) -> ()
          n237 = local write "Use mic correction"(w286) -> ()
          n238 = property on="micCorrFile" class="Path"("Value"=w285, "Visible"=w286) -> ()  [unwired: 2 in, 2 out]
          n239 = Divide(x=w287, y=2.0) -> (x/y=w290:dbl)
          n240 = property on="Fine Control" class="Slide (strict)"("Scale.Maximum"=w288, "Scale.Minimum"=w289, "Value"=w290) -> ()  [unwired: 2 in, 2 out]
        }
      }
      n241 = Empty Array?(array=w228) -> (empty?=w227:bool)
    }
  }
  n242 = while {
    tunnel: w8 -> [w487]
    stop <- w486 stop-if-true
    # "PISTONPHONE MEASUREMENT"
    n243 = Wait on Notification(notifier=w487, ignore previous (F)=TRUE) -> (notification=w485:T5, error out=w486:errorcluster)  [unwired: 2 in, 2 out]
    n244 = case shown="No Error" w486 {
      tunnel: w485 -> [w498 _]
      frame No Error {
        n245 = call "TB-Initialize Pistonphone Measurement.vi"("Exposure parameters"=w498) -> ("Params thru"=w497:T5, "error out"=w494:errorcluster)  [unwired: 13 in]
        n246 = call "AIDI-Engine.vi"("Action"=AIDI-Action."Init & Start", "error in (no error)"=w494) -> ("error out"=w493:errorcluster)  [unwired: 8 in, 5 out]
        n247 = call "AIDI-Engine.vi"("Action"=AIDI-Action."Read", "error in (no error)"=w493) -> ("AI"=w492:dbl[][], "error out"=w490:errorcluster)  [unwired: 8 in, 4 out]
        n248 = call "AIDI-Engine.vi"("Action"=AIDI-Action."Clean up", "error in (no error)"=w490) -> ("error out"=w489:errorcluster)  [unwired: 8 in, 5 out]
        n249 = case shown="No Error" w489 {
          selector: w489 -> [_ w517]
          tunnel: w492 -> [w516 _]
          tunnel: [w503 w517] -> w500
          tunnel: w497 -> [w502 _]
          frame No Error {
            n250 = Index Array(array=w516) -> (element=w512:dbl[])  [unwired: 2 in]
            "Pistonphone\nWaveform" <- w512
            n251 = call-poly <vilib>:"Mean.vi"("X"=w512) -> ("mean"=w511:dbl)  [unwired: 1 out]
            n252 = call "Range.vi"("Array"=w512) -> ("Range"=w515:dbl)
            n253 = Greater?(x=w515, y=6.0) -> (0:→"Overload":bool)
            n254 = Subtract(x=w512, y=w511) -> (x-y=w504:dbl[])
            n255 = Unbundle By Name(w502) -> ("Mic gain"=w501:dbl)
            n256 = call-poly <vilib>:"RMS.vi"("X"=w504) -> ("rms value"=w510:dbl)  [unwired: 1 out]
            n257 = local read "User ID"() -> (w505:string)
            n258 = Divide(x=w510, y=1e-06) -> (x/y=w508:dbl)
            n259 = call "Math-Linear to dB.vim"("linear"=w508) -> ("dB"=w507:dbl)
            n260 = call "TB-Save Cal Signal.vi"("Params"=w502, "ID"=w505, "Mic signal"=w504) -> ("error out"=w503:errorcluster)  [unwired: 12 in]
            n261 = Subtract(x=w507, y=w501) -> (x-y=→"Calibrator Voltage\n(dB rms re 1 uV)" →"Pistonphone Factor":dbl)
          }
          frame Error {
          }
        }
        n262 = call "Error Handler.vi"("error in (no error)"=w500) -> ("error?"=w499:bool)  [unwired: 12 in, 2 out]
        n263 = flat-sequence {
          tunnel: w499 -> [_]
          frame #0 {
            n264 = property on="Next" class="Bool"("Visible"=TRUE) -> ()  [unwired: 2 in, 2 out]
          }
        }
      }
      frame Error {
      }
    }
  }
  n265 = disable-structure shown="RUN_TIME_ENGINE==True" {
    disable-tunnel: w7 -> [w519 _]
    frame condition #0 {
      n266 = Quit LabVIEW(quit? (T)=w519) -> ()
    }
    frame condition #1 (active) {
    }
  }
